vi "Configure Trigger Source.vi"   [LabVIEW 2017, in "Agilent 6000 Series.lvlib"]
doc: "This polymorphic VI contens all trigger subVIs. You should the subVI defined by ag6000a Configure Trigger.vi."
uses:
  <instrlib>/Agilent 6000 Series/Agilent 6000 Series.lvlib
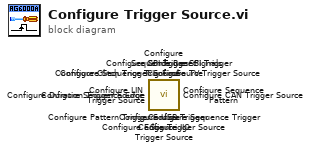
[diagram p0: block diagram]
diagram:
  n1 = call <instrlib>:"Configure USB Trigger Source.vi"() -> ()  [unwired: 14 in, 2 out]
  n2 = call <instrlib>:"Configure SPI Trigger Source.vi"() -> ()  [unwired: 14 in, 2 out]
  n3 = call <instrlib>:"Configure Sequence Edge.vi"() -> ()  [unwired: 14 in, 2 out]
  n4 = call <instrlib>:"Configure Sequence Pattern.vi"() -> ()  [unwired: 14 in, 2 out]
  n5 = call <instrlib>:"Configure Sequence Trig Find.vi"() -> ()  [unwired: 14 in, 2 out]
  n6 = call <instrlib>:"Configure Sequence Reset.vi"() -> ()  [unwired: 14 in, 2 out]
  n7 = call <instrlib>:"Configure Sequence Trigger.vi"() -> ()  [unwired: 14 in, 2 out]
  n8 = call <instrlib>:"Configure LIN Trigger Source.vi"() -> ()  [unwired: 14 in, 2 out]
  n9 = call <instrlib>:"Configure IIC Trigger Source.vi"() -> ()  [unwired: 14 in, 2 out]
  n10 = call <instrlib>:"Configure CAN Trigger Source.vi"() -> ()  [unwired: 14 in, 2 out]
  n11 = call <instrlib>:"Configure Pattern Trigger Source.vi"() -> ()  [unwired: 14 in, 2 out]
  n12 = call <instrlib>:"Configure TV Trigger Source.vi"() -> ()  [unwired: 14 in, 2 out]
  n13 = call <instrlib>:"Configure SPI Trigger Signals.vi"() -> ()  [unwired: 14 in, 2 out]
  n14 = call <instrlib>:"Configure Edge Trigger Source.vi"() -> ()  [unwired: 14 in, 2 out]
  n15 = call <instrlib>:"Configure Duration Trigger Source.vi"() -> ()  [unwired: 14 in, 2 out]
  n16 = call <instrlib>:"Configure Glitch Trigger Source.vi"() -> ()  [unwired: 14 in, 2 out]
